vi "8 PulseGenerations f+DC.vi"(8 "PulseGen Packets":u64[](array[numeric])=[0, 0, 0, 0, 0, 0, 0, 0]) -> (2 "PWMs":bool[](array[boolean]))   [LabVIEW 2014]
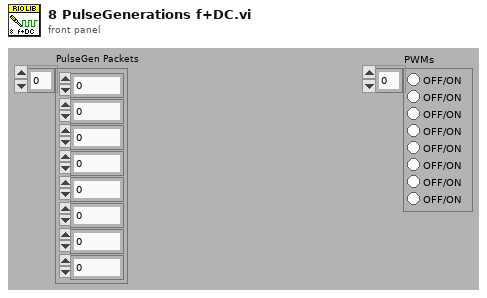
[diagram p1: front panel]
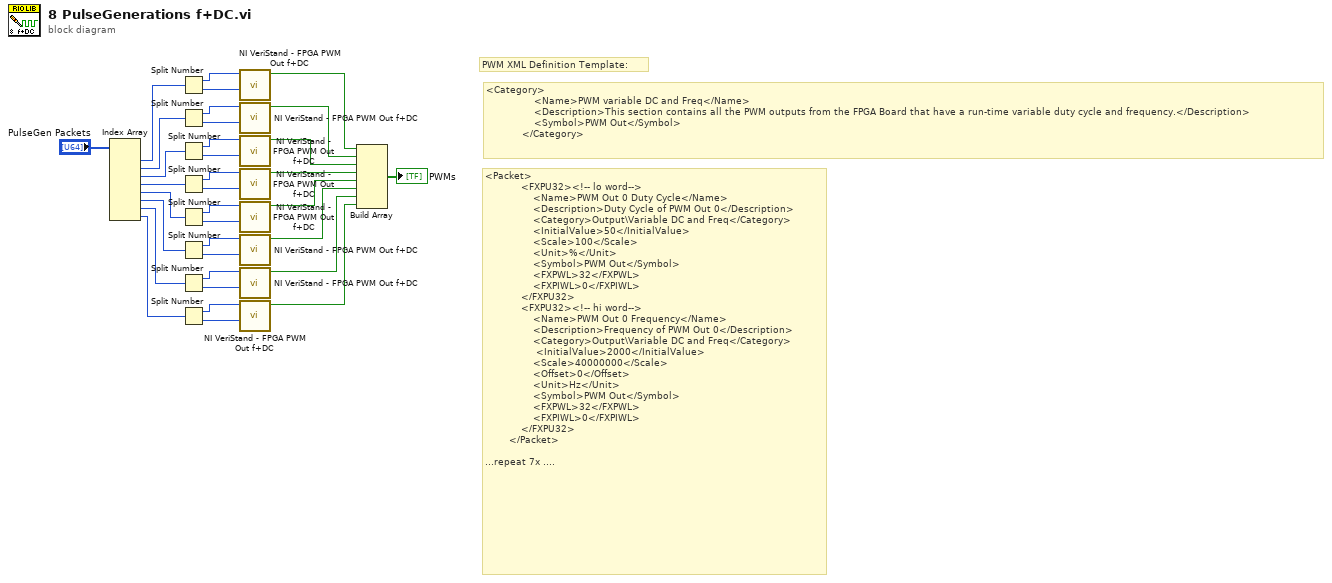
[diagram p0: block diagram]
diagram:
  # "<Category>\n                <Name>PWM variable DC and Freq</Name>\n                <Description>This section contains all the PWM outputs from the FPGA Board that have a run-time variable duty cycle and frequency.</Description>\n                <Symbol>PWM Out</Symbol>\n            </Category>"
  # "PWM XML Definition Template:"
  # "<Packet>\n            <FXPU32><!-- lo word-->\n                <Name>PWM Out 0 Duty Cycle</Name>\n                <Description>Duty Cycle of PWM Out 0</Description>\n                <Category>Output\\Variable DC and Freq</Category>\n                <InitialValue>50</InitialValue>\n\t\t\t\t            <Scale>100</Scale>\n\t\t\t            \t<Unit>%</Unit>\n                <Symbol>PWM Out</Symbol>\n\t\t\t\t            <FXPWL>32</FXPWL>\n                <FXPIWL>0</FXPIWL>\n            </FXPU32>\n            <FXPU32><!-- hi word-->\n                <Name>PWM Out 0 Frequency</Name>\n                <Description>Frequency of PWM Out 0</Description>\n                <Category>Output\\Variable DC and Freq</Category>\n\t\t\t\t             <InitialValue>2000</InitialValue>\n                <Scale>40000000</Scale>\n                <Offset>0</Offset>\n\t\t\t\t            <Unit>Hz</Unit>\n                <Symbol>PWM Out</Symbol>\n\t\t\t\t            <FXPWL>32</FXPWL>\n                <FXPIWL>0</FXPIWL>\n            </FXPU32>\n        </Packet>\n\n...repeat 7x ...."
  n1 = Index Array(array="PulseGen Packets") -> (element #1=w27:u64, element #2=w28:u64, element #3=w29:u64, element #4=w34:u64, element #5=w33:u64, element #6=w32:u64, element #7=w31:u64, element #8=w30:u64)  [unwired: 8 in]
  n2 = Split Number(x=w27) -> (hi(x)=w10:u32, lo(x)=w11:u32)
  n3 = Split Number(x=w28) -> (hi(x)=w13:u32, lo(x)=w12:u32)
  n4 = Split Number(x=w29) -> (hi(x)=w14:u32, lo(x)=w15:u32)
  n5 = Split Number(x=w34) -> (hi(x)=w17:u32, lo(x)=w16:u32)
  n6 = Split Number(x=w33) -> (hi(x)=w18:u32, lo(x)=w19:u32)
  n7 = Split Number(x=w32) -> (hi(x)=w21:u32, lo(x)=w20:u32)
  n8 = Split Number(x=w31) -> (hi(x)=w22:u32, lo(x)=w23:u32)
  n9 = Split Number(x=w30) -> (hi(x)=w25:u32, lo(x)=w24:u32)
  n10 = call "NI VeriStand - FPGA PWM Out f+DC.vi"("Duty Cycle"=w11, "Frequency"=w10) -> ("Output"=w9:bool)  [unwired: 9 in]
  n11 = call "NI VeriStand - FPGA PWM Out f+DC.vi"("Duty Cycle"=w12, "Frequency"=w13) -> ("Output"=w8:bool)  [unwired: 9 in]
  n12 = call "NI VeriStand - FPGA PWM Out f+DC.vi"("Duty Cycle"=w15, "Frequency"=w14) -> ("Output"=w7:bool)  [unwired: 9 in]
  n13 = call "NI VeriStand - FPGA PWM Out f+DC.vi"("Duty Cycle"=w16, "Frequency"=w17) -> ("Output"=w6:bool)  [unwired: 9 in]
  n14 = call "NI VeriStand - FPGA PWM Out f+DC.vi"("Duty Cycle"=w19, "Frequency"=w18) -> ("Output"=w5:bool)  [unwired: 9 in]
  n15 = call "NI VeriStand - FPGA PWM Out f+DC.vi"("Duty Cycle"=w20, "Frequency"=w21) -> ("Output"=w4:bool)  [unwired: 9 in]
  n16 = call "NI VeriStand - FPGA PWM Out f+DC.vi"("Duty Cycle"=w23, "Frequency"=w22) -> ("Output"=w3:bool)  [unwired: 9 in]
  n17 = call "NI VeriStand - FPGA PWM Out f+DC.vi"("Duty Cycle"=w24, "Frequency"=w25) -> ("Output"=w2:bool)  [unwired: 9 in]
  n18 = Build Array(w9, w8, w7, w6, w5, w4, w3, w2) -> (→"PWMs":bool[])
